vi "variables_globales.vi"() -> ()   [LabVIEW 2018]
panel:
  out "tercer_valor":dbl
  out "segundo_valor":dbl
  out "tercerproceso":string
  out "segundoproceso":string
  out "primer_valor":dbl
  out "primerproceso":string
  out "todalatrama":string
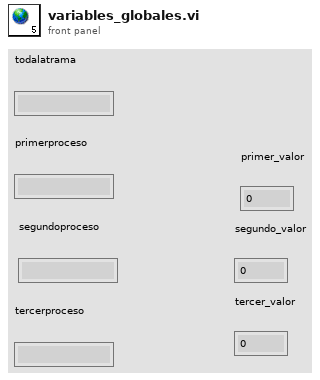
[diagram p1: front panel]
diagram:
